vi "Unflatten TreeMap from string backwards compatible.vi"(8 "error in (no error)":errorcluster, 11 "Flattened TreeMap":string) -> (0 "error out":errorcluster, 2 "version number":i32, 3 "BlueTreeMap":T1)   [LabVIEW 2020, in "Blue Tree Map OpenSource.lvlib"]
uses:
  Blue Tree Map OpenSource.lvlib
  Typedefs/Tree Map Handle.ctl
  Typedefs/Tree Map.ctl
  Typedefs/Tree Map Data.ctl
  Typedefs/Tree Node Data.ctl
  Typedefs/Attribute Map.ctl
  Typedefs/TreeMap V1.ctl
  TreeMap V1 to V2 recurse.vi
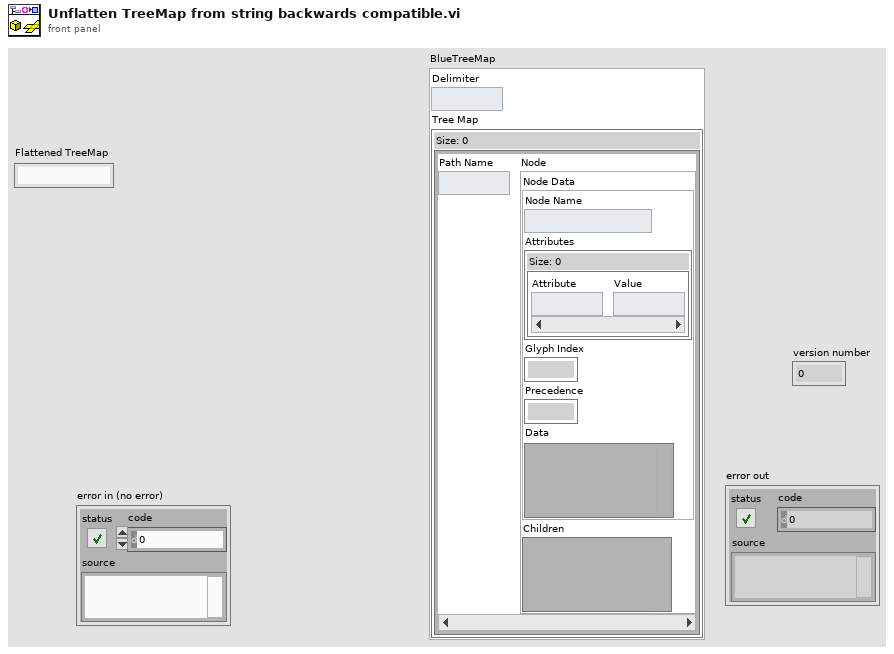
[diagram p1: front panel]
types:
  T1 = typedef "Blue Tree Map OpenSource.lvlib/Tree Map Handle.ctl" = cluster{"Delimiter":string, "Tree Map":T2}
  T2 = typedef "Blue Tree Map OpenSource.lvlib/Tree Map.ctl" = map{string, T3}
  T3 = typedef "Blue Tree Map OpenSource.lvlib/Tree Map Data.ctl" = cluster{"Node Data":T4, "Children":variant}
  T4 = typedef "Blue Tree Map OpenSource.lvlib/Tree Node Data.ctl" = cluster{"Node Name":string, "Attributes":T5, "Glyph Index":i32, "Precedence":i32, "Data":variant}
  T5 = typedef "Blue Tree Map OpenSource.lvlib/Attribute Map.ctl" = map{string, string}
  T6 = typedef "Blue Tree Map OpenSource.lvlib/TreeMap V1.ctl" = cluster{"Delimiter":string, "Tree Map":map{string, cluster{"Node Data":cluster{"Node Name":string, "Attributes":T5, "Glyph Index":i32, "Precedence":i32}, "Children":variant}}}
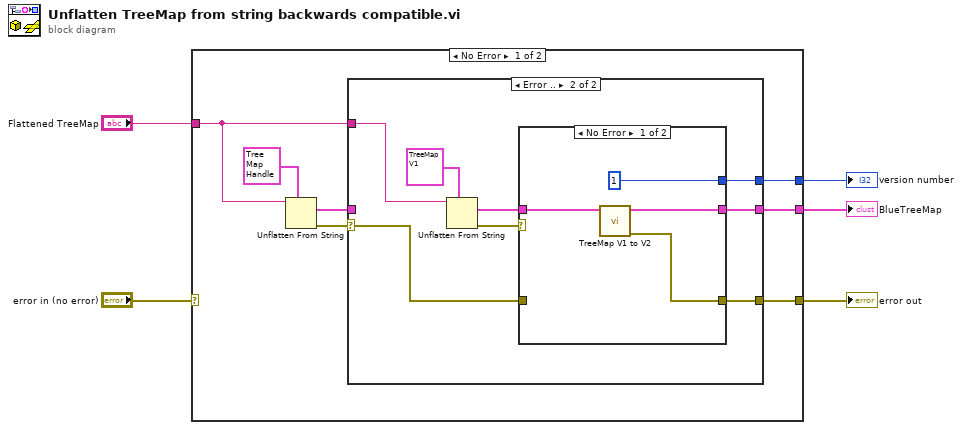
[diagram p0: block diagram]
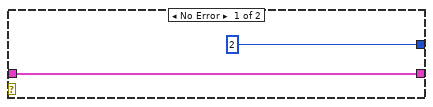
[diagram p2: hidden frame]
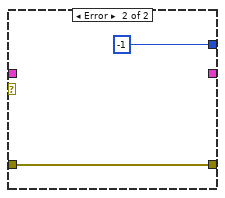
[diagram p3: hidden frame]
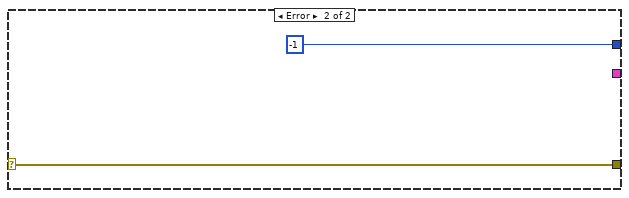
[diagram p4: hidden frame]
diagram:
  n1 = case shown="No Error" "error in (no error)" {
    selector: "error in (no error)" -> [_ w30]
    tunnel: "Flattened TreeMap" -> [w10 _]
    tunnel: [w8 _] -> w3
    tunnel: [w7 w30] -> w2
    tunnel: [w6 -1 ("version number")] -> w1
    frame No Error {
      n2 = Unflatten From String(type=T1 {"Delimiter"="", "Tree Map"={}} ("BlueTreeMap"), binary string=w10) -> (value=w9:T1, error out=w11:errorcluster)  [unwired: 3 in, 1 out]
      n3 = case shown="Error .." w11 {
        selector: w11 -> [_ w16]
        tunnel: w10 -> [_ w22]
        tunnel: w9 -> [w14 _]
        tunnel: [w14 w18] -> w8
        tunnel: [_ w17] -> w7
        tunnel: [2 ("version number") w15] -> w6
        frame No Error {
        }
        frame Error {
          n4 = Unflatten From String(type=T6 {"Delimiter"="", "Tree Map"={}} ("V1"), binary string=w22) -> (value=w19:T6, error out=w20:errorcluster)  [unwired: 3 in, 1 out]
          n5 = case shown="No Error" w20 {
            tunnel: w19 -> [w25 _]
            tunnel: [w26 _] -> w18
            tunnel: [w24 w28] -> w17
            tunnel: w16 -> [_ w28]
            tunnel: [1 ("version number") -1 ("version number")] -> w15
            frame No Error {
              n6 = call "TreeMap V1 to V2.vi"("V1"=w25) -> ("error out"=w24:errorcluster, "V2"=w26:T1)  [unwired: 9 in]
            }
            frame Error {
            }
          }
        }
      }
    }
    frame Error {
    }
  }
  "error out" <- w2
  "BlueTreeMap" <- w3
  "version number" <- w1
